vi "Resize.vi"(0 "reference in":refnum<class "RectangularNode.lvclass">, 1 "dx":dbl format="%.2f", 2 "dy":dbl format="%.2f", 3 "Positions":T1, 5 "error in (no error)":errorcluster) -> (14 "reference out":refnum<class "RectangularNode.lvclass">, 19 "error out":errorcluster)   [LabVIEW 2014, in "RectangularNode.lvclass"]
uses:
  <resource>/Framework/Providers/Open_GDS/UML/RectangularNode_class/RectangularNode.lvclass
  <resource>/Framework/Providers/Open_GDS/UML/UMLEditor/UMLEditor_HotSpotType.ctl
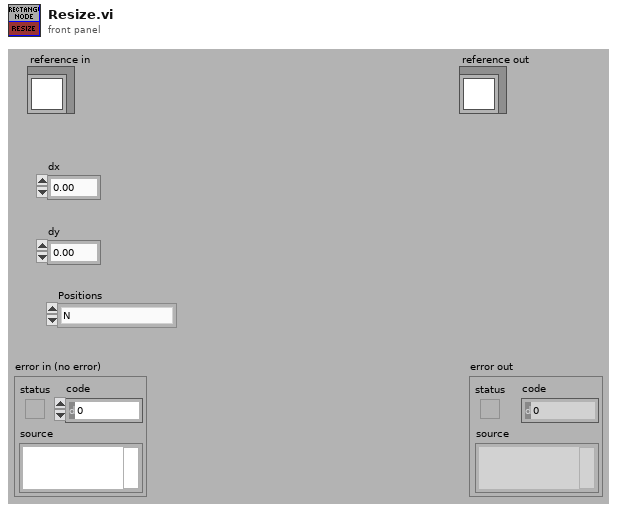
[diagram p1: front panel]
types:
  T1 = typedef "UMLEditor_HotSpotType.ctl" = enum16{"N", "NE", "E", "SE", "S", "SW", "W", "NW", "Expand", "Collaps"}
  T2 = typedef "RectangularNode.lvclass/ObjectAttributes.ctl" = cluster{"bounds":T3}
  T3 = typedef "Rectangle Rectangle2D.ctl" = cluster{"x":dbl, "y":dbl, "width":dbl, "height":dbl}
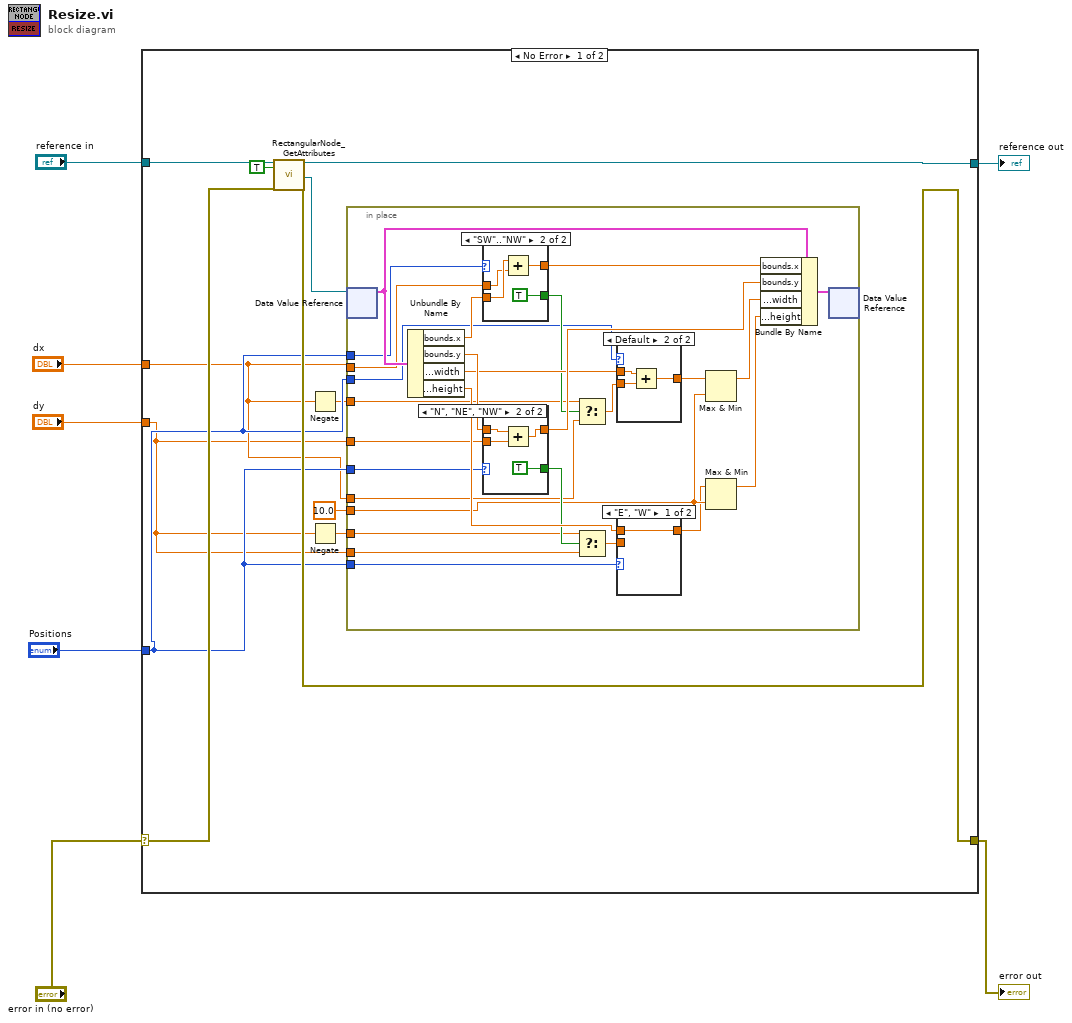
[diagram p0: block diagram]
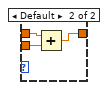
[diagram p2: hidden frame]
diagram:
  n1 = case shown="No Error" "error in (no error)" {
    selector: "error in (no error)" -> [w17 w66]
    tunnel: [w19 w66] -> w6
    tunnel: [w16 w65] -> w4
    tunnel: "reference in" -> [w18 w65]
    tunnel: "dx" -> [w11 _]
    tunnel: "dy" -> [w9 _]
    tunnel: "Positions" -> [w12 _]
    frame No Error {
      n2 = call <resource>:"RectangularNode_GetAttributes.vi"("reference in"=w18, "OnlyGetDvrReference(False)"=TRUE, "error in (no error)"=w17) -> ("reference out"=w16:refnum<class "RectangularNode.lvclass">, "DataRef"=w14:refnum<data-value>, "error out"=w19:errorcluster)  [unwired: 13 in, 1 out]
      n3 = Negate(x=w11) -> (-x=w10:dbl)
      n4 = Negate(x=w9) -> (-x=w8:dbl)
      n5 = in-place {
        in-place-border: w12 -> [w36]
        in-place-border: w11 -> [w35]
        in-place-border: w12 -> [w33]
        in-place-border: w9 -> [w32]
        in-place-border: 10.0 ("y") -> [w29]
        in-place-border: w12 -> [w27]
        in-place-border: w12 -> [w25]
        in-place-border: w11 -> [w23]
        in-place-border: w10 -> [w22]
        in-place-border: w9 -> [w21]
        in-place-border: w8 -> [w20]
        n6 = in-place-dvr #1(w14) -> (w46:T2)  [unwired: 1 out]
        n7 = Unbundle By Name(w46) -> ("bounds.x"=w40:dbl, "bounds.y"=w39:dbl, "bounds.width"=w38:dbl, "bounds.height"=w37:dbl)
        n8 = case shown="\"SW\"..\"NW\"" w36 {
          tunnel: w40 -> [w60 w64]
          tunnel: [w60 w63] -> w45
          tunnel: w35 -> [_ w62]
          tunnel: [_ TRUE] -> w34
          frame Default {
          }
          frame "SW".."NW" {
            n9 = Add(x=w64, y=w62) -> (x+y=w63:dbl)
          }
        }
        n10 = case shown="\"N\", \"NE\", \"NW\"" w33 {
          tunnel: w39 -> [w55 w59]
          tunnel: [w55 w58] -> w44
          tunnel: w32 -> [_ w57]
          tunnel: [_ TRUE] -> w31
          frame Default {
          }
          frame "N", "NE", "NW" {
            n11 = Add(x=w59, y=w57) -> (x+y=w58:dbl)
          }
        }
        n12 = Select(t=w22, s=w34, f=w23) -> (s? t:f=w26:dbl)
        n13 = Select(t=w20, s=w31, f=w21) -> (s? t:f=w24:dbl)
        n14 = case shown="Default" w27 {
          tunnel: w38 -> [w51 w54]
          tunnel: w26 -> [_ w53]
          tunnel: [w51 w52] -> w30
          frame "N", "S" {
          }
          frame Default {
            n15 = Add(x=w54, y=w53) -> (x+y=w52:dbl)
          }
        }
        n16 = case shown="\"E\", \"W\"" w25 {
          tunnel: w37 -> [w47 w50]
          tunnel: w24 -> [_ w49]
          tunnel: [w47 w48] -> w28
          frame "E", "W" {
          }
          frame Default {
            n17 = Add(x=w50, y=w49) -> (x+y=w48:dbl)
          }
        }
        n18 = Max & Min(x=w30, y=w29) -> (max(x,y)=w43:dbl)  [unwired: 1 out]
        n19 = Max & Min(x=w28, y=w29) -> (max(x,y)=w42:dbl)  [unwired: 1 out]
        n20 = Bundle By Name(cluster=w46, "bounds.x"=w45, "bounds.y"=w44, "bounds.width"=w43, "bounds.height"=w42) -> (w41:T2)
        n21 = in-place-dvr #1(w41) -> ()  [unwired: 2 out]
      }
    }
    frame Error {
    }
  }
  "error out" <- w6
  "reference out" <- w4
